vi "Measure.vi"(8 "error in (no error)":errorcluster, 11 "4300 in":refnum<class "4300.lvclass">) -> (0 "error out":errorcluster, 3 "4300 out":refnum<class "4300.lvclass">)   [LabVIEW 2019, in "4300.lvlib" / "4300.lvclass"]
uses:
  Library/4300.lvclass
  builds/Instruments/AnalogInput.lvlibp/Library/AnalogInput.lvclass
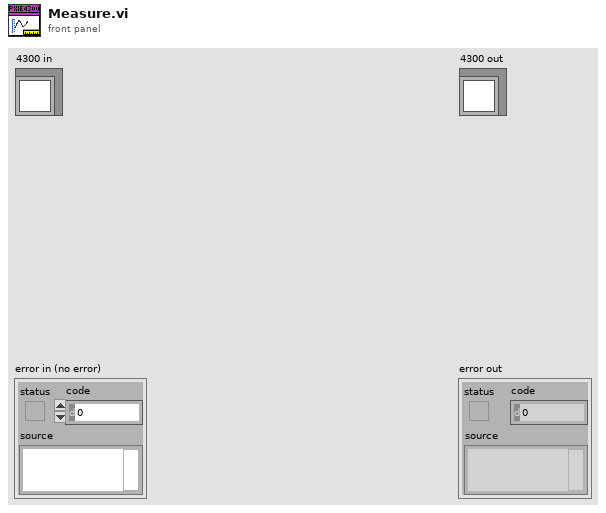
[diagram p1: front panel]
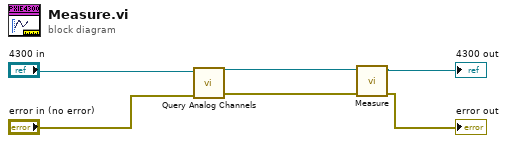
[diagram p0: block diagram]
diagram:
  n1 = call-dynamic "Query Analog Channels.vi"("error in"="error in (no error)", "4300 in"="4300 in") -> ("error out"=w2:errorcluster, "4300 out"=w3:refnum<class "4300.lvclass">)  [unwired: 7 in, 1 out]
  n2 = call-parent "Measure.vi"("error in"=w2, "AnalogInput in"=w3) -> ("error out"=→"error out":errorcluster, "AnalogInput out"=→"4300 out":refnum<class "4300.lvclass">)  [unwired: 8 in]
